vi "fpga_FIFO control (P Class).vi"(0 "Time stamp":fxp<+,64,32> format="%.42g", 1 "reset":bool, 2 "freq time difference [s]":fxp<+,18,-4>, 5 "Frequency":fxp<+,32,8>, 7 "#ch":fxp<+,5,5>, 9 "PMU VI input valid":bool, 11 "PMU VI output valid":bool) -> (4 "Time Stamp out":fxp<+,64,32> format="%.42g", 15 "Frequency output":fxp<+,32,8> format="%.27g")   [LabVIEW 2013, in "NI_EP_PMU_FPGA.lvlib"]
uses:
  <vilib>/addons/Electrical Power/PMU/NI_EP_PMU_FPGA.lvlib
  <vilib>/rvi/Emulation/niFpgaSctlEmulationGetInTimedLoop.vi
  <vilib>/rvi/DataTransferAndStorage/Container/Common/niFpgaContainerGetUniqueNameForEmu.vi
  <vilib>/rvi/DataTransferAndStorage/Container/Common/niFpgaContainerSetEmuInfo.vi
  <vilib>/rvi/eio/common/nirviEmuReportErrorAndStop.vi
  <vilib>/rvi/FIFO/Fifo_Resource/nirvififoEmulationSetSize.vi
  <vilib>/rvi/errors/niFpgaSetErrorForExecOnDevCompSimple.vi
  <vilib>/rvi/Emulation/niFpgaSctlEmulationFifoFullMgr.vi
  <vilib>/rvi/Emulation/niFpgaSctlEmulationResourceMgr.vi
  <vilib>/rvi/LocalResourceManager/LocalResourceManager.xnode
  <vilib>/rvi/DataTransferAndStorage/Container/XNode/niFpgaContainer.xnode
  <vilib>/rvi/FIFO/Fifo_Resource/nirvififoEmulationWrite.vi
  <vilib>/rvi/FXPMathLib/FxpSub/XNode/nifxpmath_Sub.xnode
  <vilib>/rvi/FXPMathLib/basic elements/FxpDiscreteDelay/XNode/nifxpmath_DiscreteDelay.xnode
  <vilib>/rvi/FIFO/Fifo_Resource/nirvififoEmulationRead.vi
  <vilib>/addons/Electrical Power/PQ/Resampling/NI_EP_Resample_FPGA.lvlib
  <vilib>/rvi/FXPMathLib/sim/FxpSim.dll
types:
  T1 = cluster{"frequency":fxp<+,32,8>, "timestamp":fxp<+,64,32>}
  T2 = cluster{"frequency":fxp<+,32,8>, "timestamp":fxp<+,64,32>}[]
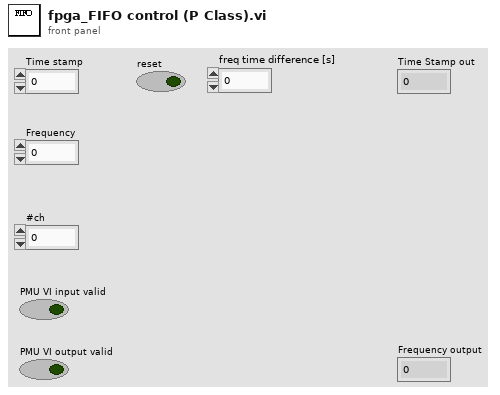
[diagram p1: front panel]
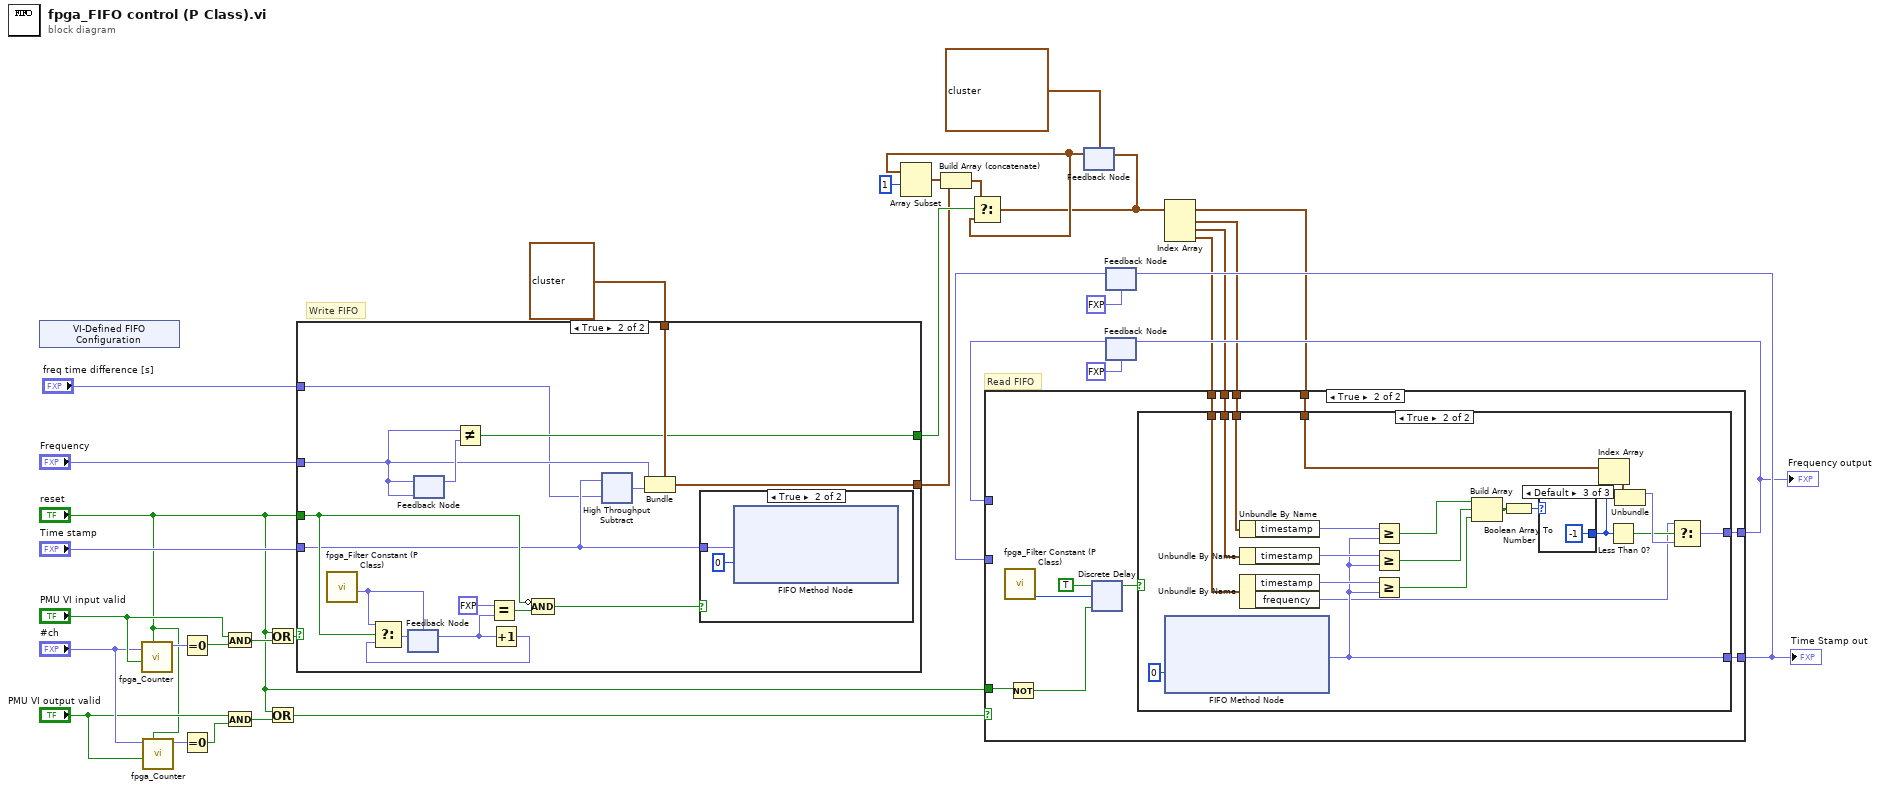
[diagram p0: block diagram]
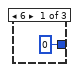
[diagram p4: hidden frame]
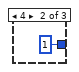
[diagram p5: hidden frame]
diagram:
  # "Read FIFO"
  # "Write FIFO"
  n1 = xnode "VI-Defined FIFO Configuration"() -> ()  [unwired: 1 out]
  n2 = call <vilib>:"fpga_Counter.vi"("reset"="reset", "Input Valid?"="PMU VI input valid", "upper limit"="#ch") -> ("count"=w20:fxp<+,5,5>)  [unwired: 7 in, 1 out]
  n3 = call <vilib>:"fpga_Counter.vi"("reset"="reset", "Input Valid?"="PMU VI output valid", "upper limit"="#ch") -> ("count"=w19:fxp<+,5,5>)  [unwired: 7 in, 1 out]
  n4 = Equal To 0?(x=w20) -> (x = 0?=w32:bool)
  n5 = Equal To 0?(x=w19) -> (x = 0?=w27:bool)
  n6 = And(x="PMU VI input valid", y=w32) -> (x .and. y?=w24:bool)
  n7 = And(x="PMU VI output valid", y=w27) -> (x .and. y?=w31:bool)
  n8 = Or(x="reset", y=w24) -> (x .or. y?=w23:bool)
  n9 = Or(x="reset", y=w31) -> (x .or. y?=w30:bool)
  n10 = case shown="True" w23 {
    tunnel: "Time stamp" -> [_ w36]
    tunnel: "reset" -> [_ w44]
    tunnel: "Frequency" -> [_ w35]
    tunnel: [_ w37] -> w11
    tunnel: [_ w39] -> w10
    tunnel: T1 {"frequency"=0.0, "timestamp"=0.0} -> [_ w38]
    tunnel: "freq time difference [s]" -> [_ w34]
    frame False {
    }
    frame True {
      n11 = call <vilib>:"fpga_Filter Constant (P Class).vi"() -> ("Start"=w43:fxp<+/-,4,4>)  [unwired: 8 in, 3 out]
      n12 = feedback #1(w43) -> (w47:fxp<+/-,4,4>)
      n13 = feedback #2(w35) -> (w41:fxp<+,32,8>)
      n14 = feedback-in #2(w35) -> ()
      n15 = Not Equal?(x=w35, y=w41) -> (x != y?=w37:bool)
      n16 = Equal?(x=fxp<+/-,4,4> 4.0, y=w47) -> (x = y?=w45:bool)
      n17 = Increment(x=w47) -> (x+1=w48:fxp<+,3,3>)
      n18 = Select(t=w43, s=w44, f=w48) -> (s? t:f=w49:fxp<+/-,4,4>)
      n19 = feedback-in #1(w49) -> ()
      n20 = Compound Arithmetic op=AND(invert w44, w45) -> (w42:bool)
      n21 = xnode "High Throughput Subtract"("x"=w36, "y"=w34) -> ("x-y"=w40:fxp<+,64,32>)
      n22 = Bundle(cluster=w38, "frequency"=w35, "timestamp"=w40) -> (w39:T1)
      n23 = case shown="True" w42 {
        tunnel: w36 -> [_ w50]
        frame False {
        }
        frame True {
          n24 = xnode ("FIFO Method Node")("Element"=w50, "Timeout"=0) -> ()  [unwired: 1 in, 2 out]
        }
      }
    }
  }
  n25 = feedback #3(T2 [{"frequency"=0.0, "timestamp"=0.0}, {"frequency"=0.0, "timestamp"=0.0}, {"frequency"=0.0, "timestamp"=0.0}]) -> (w6:T2)
  n26 = Array Subset(array=w6, index=1) -> (w12:T2)  [unwired: 1 in]
  n27 = Build Array (concatenate)(w12, w10) -> (w7:T2)
  n28 = Select(t=w7, s=w11, f=w6) -> (s? t:f=w1:T2)
  n29 = feedback-in #3(w1) -> ()
  n30 = feedback #4(fxp<+,64,32> 0.0 ("Element")) -> (w28:fxp<+,64,32>)
  n31 = feedback #5(fxp<+,32,8> 0.0 ("Element")) -> (w25:fxp<+,32,8>)
  n32 = Index Array(array=w1) -> (element #1=w4:T1, element #2=w3:T1, element #3=w2:T1)  [unwired: 3 in]
  n33 = case shown="True" w30 {
    tunnel: "reset" -> [_ w62]
    tunnel: [w53 w64] -> w29
    tunnel: w28 -> [w53 _]
    tunnel: [w52 w63] -> w15
    tunnel: w25 -> [w52 _]
    tunnel: w4 -> [_ w57]
    tunnel: w1 -> [_ w56]
    tunnel: w3 -> [_ w55]
    tunnel: w2 -> [_ w54]
    frame False {
    }
    frame True {
      n34 = call <vilib>:"fpga_Filter Constant (P Class).vi"() -> ("Total Delay"=w58:u8)  [unwired: 8 in, 3 out]
      n35 = Not(x=w62) -> (.not. x?=w60:bool)
      n36 = xnode ("Discrete Delay")("D"=TRUE, "n-1[0..255]"=w58, "enable"=w60) -> ("Q"=w59:bool)
      n37 = case shown="True" w59 {
        tunnel: [_ w73] -> w64
        tunnel: [_ w69] -> w63
        tunnel: w57 -> [_ w83]
        tunnel: w56 -> [_ w81]
        tunnel: w55 -> [_ w78]
        tunnel: w54 -> [_ w75]
        frame False {
        }
        frame True {
          n38 = xnode ("FIFO Method Node")("Timeout"=0) -> ("Element"=w73:fxp<+,64,32>)  [unwired: 1 in, 2 out]
          n39 = Unbundle By Name(w83) -> ("timestamp"=w82:fxp<+,64,32>)
          n40 = Unbundle By Name(w78) -> ("timestamp"=w77:fxp<+,64,32>)
          n41 = Unbundle By Name(w75) -> ("timestamp"=w74:fxp<+,64,32>, "frequency"=w66:fxp<+,32,8>)
          n42 = Greater Or Equal?(x=w82, y=w73) -> (x >= y?=w65:bool)
          n43 = Greater Or Equal?(x=w77, y=w73) -> (x >= y?=w76:bool)
          n44 = Greater Or Equal?(x=w74, y=w73) -> (x >= y?=w72:bool)
          n45 = Build Array(w65, w76, w72) -> (w80:bool[])
          n46 = Boolean Array To Number(Boolean array=w80) -> (number=w67:u8)
          n47 = case shown="Default" w67 {
            tunnel: [0 ("index") 1 ("index") -1 ("index")] -> w71
            frame 6 {
            }
            frame 4 {
            }
            frame Default {
            }
          }
          n48 = Index Array(array=w81, index=w71) -> (element=w79:T1)
          n49 = Less Than 0?(x=w71) -> (x < 0?=w68:bool)
          n50 = Unbundle(w79) -> ("frequency"=w70:fxp<+,32,8>)  [unwired: 1 out]
          n51 = Select(t=w66, s=w68, f=w70) -> (s? t:f=w69:fxp<+,32,8>)
        }
      }
    }
  }
  "Time Stamp out" <- w29
  "Frequency output" <- w15
  n52 = feedback-in #4(w29) -> ()
  n53 = feedback-in #5(w15) -> ()
